vi "Read Pulse.vi"(8 "error in (no error)":errorcluster, 9 "Pulse (1: Transition 1)":i32(ring)=1 items=["Transition 1"=1, "Transition 2"=2, "Transition 3"=3, "Transition 4"=4, "Transition 5"=5, "Transition 6"=6, "Transition 7"=7, "Transition 8"=8, "Transition 9"=9, "Transition 10"=10, "Transition 11"=11, "Transition 12"=12, "Transition 13"=13, "Transition 14"=14, "Transition 15"=15, "Transition 16"=16, "Transition 17"=17, "Transition 18"=18, "Transition 19"=19, "Transition 20"=20], 11 "VISA resource name":refnum<visa-resource-name>) -> (0 "error out":errorcluster, 1 "Duration":dbl, 2 "Duty Cycle":dbl, 3 "VISA resource name out":refnum<visa-resource-name>, 4 "Separation":dbl, 5 "Period":dbl)   [LabVIEW 2014, in "Agilent U2000 Series.lvlib"]
doc: "Returns the data related to power pulses.\n\nNote: \n(1) If the free-run trigger acquisition is selected, error -221, \"Settings conflict\" occurs.\n(2) This function supports model U2020 X-Series and U2042XA/U2044XA/U2049XA only."
uses:
  Agilent U2000 Series.lvlib
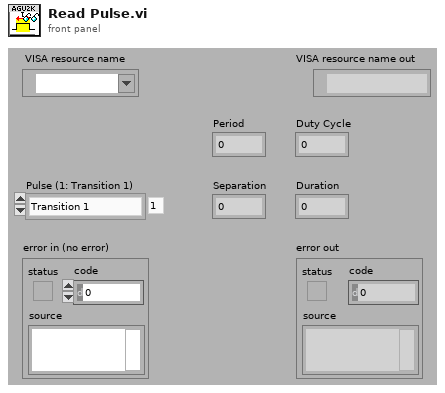
[diagram p1: front panel]
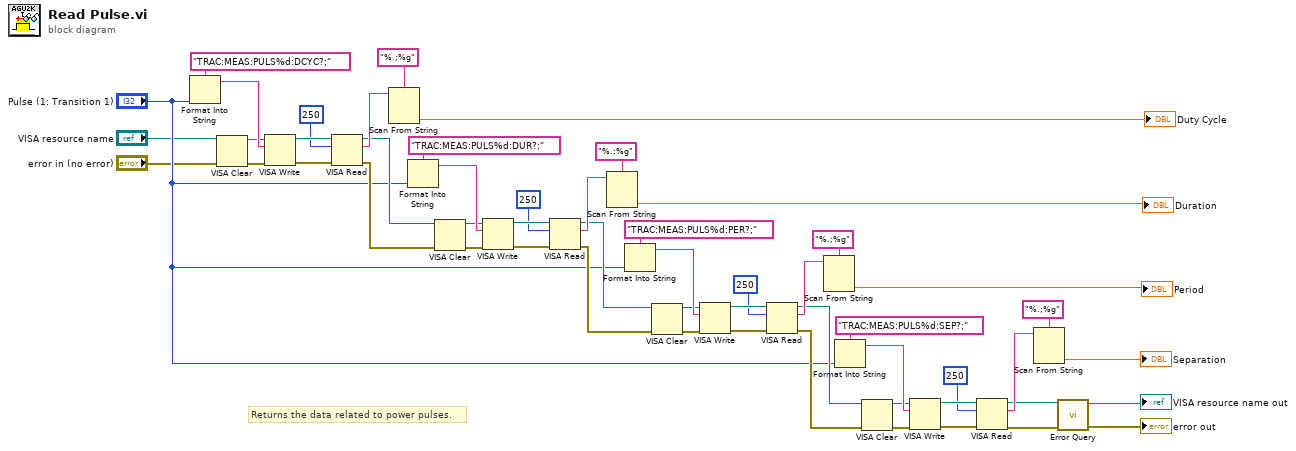
[diagram p0: block diagram]
diagram:
  # "Returns the data related to power pulses."
  n1 = Format Into String(format string="TRAC:MEAS:PULS%d:DCYC?;", "Pulse (1: Transition 1)") -> (resulting string=w24:string)  [unwired: 2 in, 1 out]
  n2 = VISA Clear(VISA resource name="VISA resource name", error in (no error)="error in (no error)") -> (VISA resource name out=w18:refnum<visa-resource-name>, error out=w17:errorcluster)
  n3 = VISA Write(VISA resource name=w18, write buffer=w24, error in (no error)=w17) -> (VISA resource name out=w22:refnum<visa-resource-name>, error out=w23:errorcluster)  [unwired: 1 out]
  n4 = VISA Read(VISA resource name=w22, byte count=u32 250, error in (no error)=w23) -> (VISA resource name out=w12:refnum<visa-resource-name>, read buffer=w20:string, error out=w11:errorcluster)  [unwired: 1 out]
  n5 = Scan From String(format string="%.;%g", input string=w20) -> (output 1=→"Duty Cycle":dbl)  [unwired: 2 in, 4 out]
  n6 = Format Into String(format string="TRAC:MEAS:PULS%d:DUR?;", "Pulse (1: Transition 1)") -> (resulting string=w33:string)  [unwired: 2 in, 1 out]
  n7 = VISA Clear(VISA resource name=w12, error in (no error)=w11) -> (VISA resource name out=w27:refnum<visa-resource-name>, error out=w26:errorcluster)
  n8 = VISA Write(VISA resource name=w27, write buffer=w33, error in (no error)=w26) -> (VISA resource name out=w31:refnum<visa-resource-name>, error out=w32:errorcluster)  [unwired: 1 out]
  n9 = VISA Read(VISA resource name=w31, byte count=u32 250, error in (no error)=w32) -> (VISA resource name out=w14:refnum<visa-resource-name>, read buffer=w29:string, error out=w13:errorcluster)  [unwired: 1 out]
  n10 = Scan From String(format string="%.;%g", input string=w29) -> (output 1=→"Duration":dbl)  [unwired: 2 in, 4 out]
  n11 = Format Into String(format string="TRAC:MEAS:PULS%d:PER?;", "Pulse (1: Transition 1)") -> (resulting string=w42:string)  [unwired: 2 in, 1 out]
  n12 = VISA Clear(VISA resource name=w14, error in (no error)=w13) -> (VISA resource name out=w36:refnum<visa-resource-name>, error out=w35:errorcluster)
  n13 = VISA Write(VISA resource name=w36, write buffer=w42, error in (no error)=w35) -> (VISA resource name out=w40:refnum<visa-resource-name>, error out=w41:errorcluster)  [unwired: 1 out]
  n14 = VISA Read(VISA resource name=w40, byte count=u32 250, error in (no error)=w41) -> (VISA resource name out=w16:refnum<visa-resource-name>, read buffer=w38:string, error out=w15:errorcluster)  [unwired: 1 out]
  n15 = Scan From String(format string="%.;%g", input string=w38) -> (output 1=→"Period":dbl)  [unwired: 2 in, 4 out]
  n16 = Format Into String(format string="TRAC:MEAS:PULS%d:SEP?;", "Pulse (1: Transition 1)") -> (resulting string=w52:string)  [unwired: 2 in, 1 out]
  n17 = VISA Clear(VISA resource name=w16, error in (no error)=w15) -> (VISA resource name out=w45:refnum<visa-resource-name>, error out=w44:errorcluster)
  n18 = VISA Write(VISA resource name=w45, write buffer=w52, error in (no error)=w44) -> (VISA resource name out=w50:refnum<visa-resource-name>, error out=w51:errorcluster)  [unwired: 1 out]
  n19 = VISA Read(VISA resource name=w50, byte count=u32 250, error in (no error)=w51) -> (VISA resource name out=w4:refnum<visa-resource-name>, read buffer=w48:string, error out=w1:errorcluster)  [unwired: 1 out]
  n20 = Scan From String(format string="%.;%g", input string=w48) -> (output 1=→"Separation":dbl)  [unwired: 2 in, 4 out]
  n21 = call "Error Query.vi"("error in (no error)"=w1, "VISA resource name"=w4) -> ("error out"=→"error out":errorcluster, "VISA resource name out"=→"VISA resource name out":refnum<visa-resource-name>)  [unwired: 8 out]
